vi "AlarmEngineModule.vi"(8 "error in (no error)":errorcluster, 9 "Shutdown Event":refnum<user-event>, 10 "Config":T1, 11 "ModuleID":string) -> (0 "error out":errorcluster)   [LabVIEW 2020, in "AlarmEngine.lvlib"]
uses:
  AlarmEngine.lvlib
  <vilib>/Utility/Data Type/Type Definitions/Data Type.ctl
  <vilib>/Utility/Data Type/NI_Data Type.lvlib
  eac3c09b-8ce1-4b18-8db3-0e6b686db002.vi
  <vilib>/Tag Engine/Types/SetRequest Cluster.ctl
  <vilib>/Tag Engine/Tag Engine Core.lvlib
  <vilib>/Tag Engine/Tag Expr/Tag Expr.lvclass
  fca5b91c-2f04-4d42-a9b6-24fda182e91a.vi
  cc66a33a-e2f7-4f32-842c-e417093018b7.vi
  <vilib>/Tag Engine/Tag/Tag.lvclass
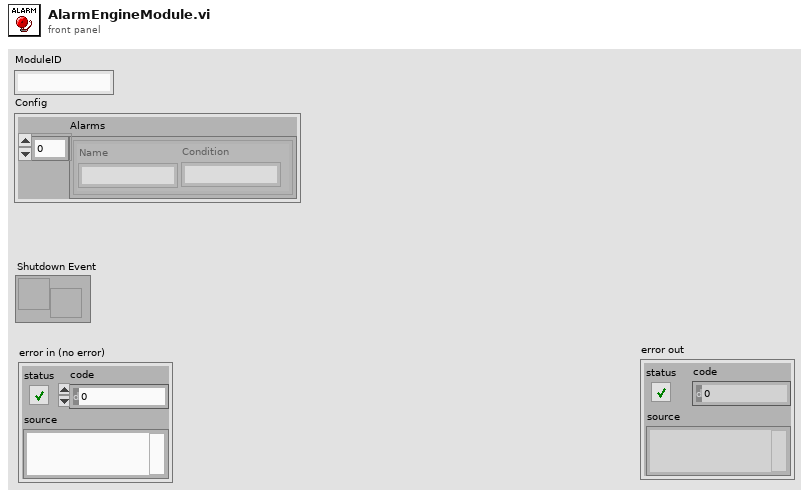
[diagram p1: front panel]
types:
  T1 = cluster{"Alarms":cluster{"Name":string, "Condition":string}[]}
  T2 = cluster{"Tag Refs":cluster{"ALARMS":refnum<data-value>[], "CONFIG":refnum<data-value>}, "Config":cluster{"Alarms":cluster{"Name":string, "Condition":string}[]}, "Conditions":refnum<class "Tag Expr.lvclass">[]}
  T3 = cluster{"ALARMS":refnum<data-value>[], "CONFIG":refnum<data-value>}
  T4 = cluster{"Config":cluster{"Alarms":cluster{"Name":string, "Condition":string}[]}, "Callback":refnum<notifier>}
  T5 = cluster{"Req Value":variant, "Callback":refnum<notifier>}
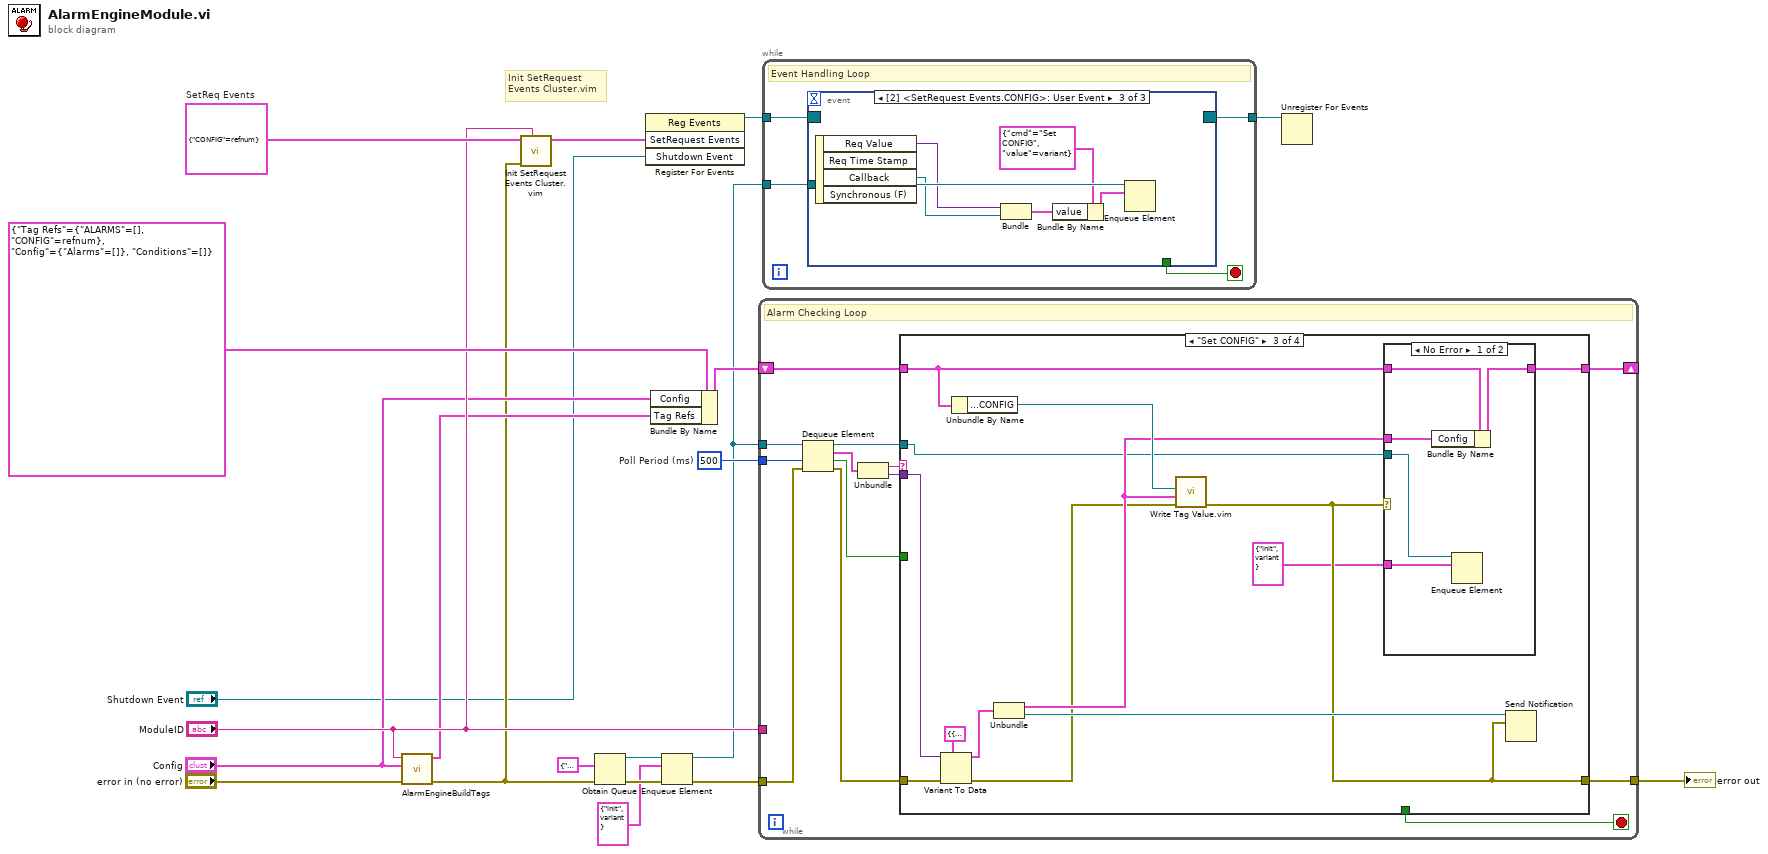
[diagram p0: block diagram]
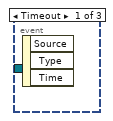
[diagram p2: hidden frame]
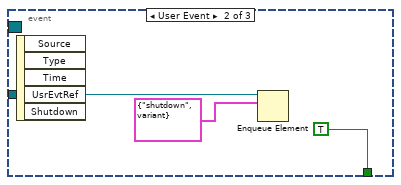
[diagram p3: hidden frame]
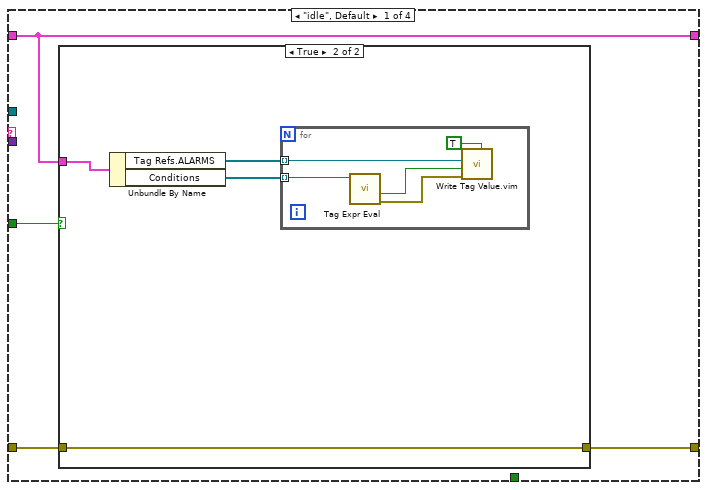
[diagram p4: hidden frame]
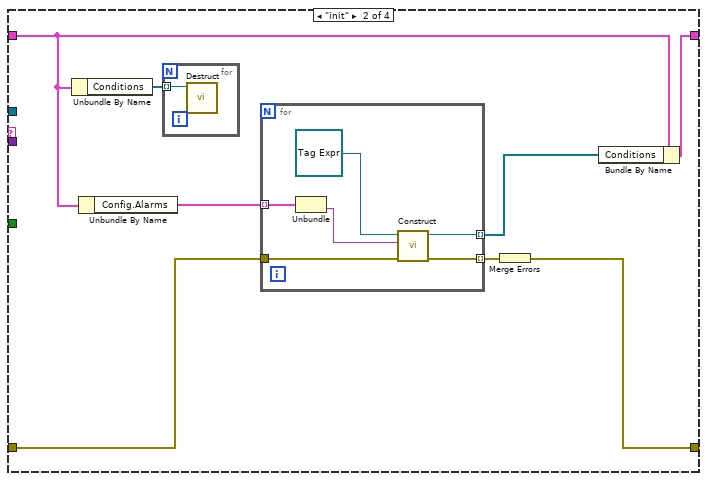
[diagram p6: hidden frame]
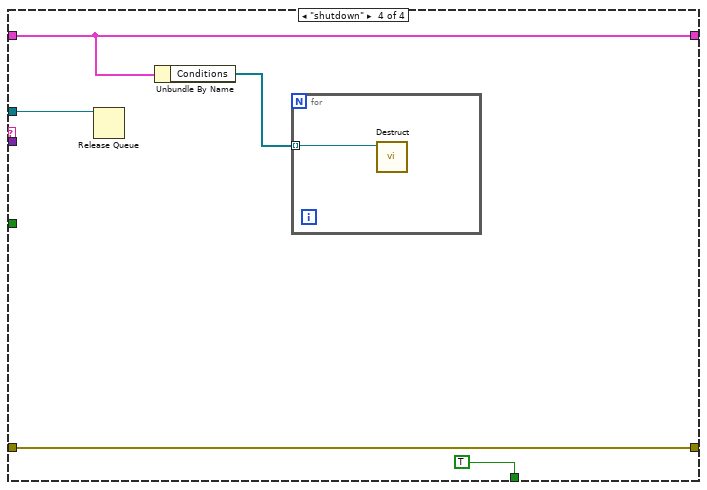
[diagram p8: hidden frame]
diagram:
  w7 = 500  # Poll Period (ms)
  w18 = cluster{"CONFIG":refnum<user-event>} {"CONFIG"=refnum}  # SetReq Events
  # "Init SetRequest\nEvents Cluster.vim"
  n1 = call "AlarmEngineBuildTags.vi"("error in (no error)"="error in (no error)", "Config"="Config", "ModuleID"="ModuleID") -> ("error out"=w9:errorcluster, "Tag Refs"=w10:T3)  [unwired: 7 in]
  n2 = call "Init SetRequest Events Cluster.vim"("Namespace"="ModuleID", "error in (no error)"=w9, "SetRequest Events in"=w18) -> ("SetRequest Events"=w17:cluster{"CONFIG":refnum<user-event>})  [unwired: 7 in, 1 out]
  n3 = Obtain Queue(element data type=cluster{"cmd":string, "value":variant} {"cmd"="", "value"=variant}, error in (no error)=w9) -> (queue out=w5:refnum<queue>, error out=w4:errorcluster)  [unwired: 3 in, 1 out]
  n4 = register-events(w17, "Shutdown Event") -> (reference out=w19:refnum<event-registration>)  [unwired: 2 in, 1 out]
  n5 = Bundle By Name(cluster=T2 {"Tag Refs"={"ALARMS"=[], "CONFIG"=refnum}, "Config"={"Alarms"=[]}, "Conditions"=[]}, "Config"="Config", "Tag Refs"=w10) -> (w8:T2)
  n6 = Enqueue Element(queue=w5, element=cluster{"cmd":string, "value":variant} {"cmd"="init", "value"=variant}, error in (no error)=w4) -> (queue out=w1:refnum<queue>, error out=w2:errorcluster)  [unwired: 1 in, 1 out]
  n7 = while {
    tunnel: "ModuleID" -> [_]
    tunnel: w2 -> [w33]
    shift-right: [w25] -> _
    shift-left: w8 -> [w32]
    tunnel: w1 -> [w29]
    tunnel: [w23] -> w15
    tunnel: w7 -> [w21]
    stop <- w24 stop-if-true
    # "Alarm Checking Loop"
    n8 = Dequeue Element(queue=w29, timeout in ms (-1)=w21, error in (no error)=w33) -> (queue out=w30:refnum<queue>, element=w28:cluster{"cmd":string, "value":variant}, timed out?=w22:bool, error out=w31:errorcluster)
    n9 = Unbundle(w28) -> ("cmd"=w27:string, "value"=w26:variant)
    n10 = case shown="\"Set CONFIG\"" w27 {
      tunnel: w32 -> [w37 w52 w66 w83]
      tunnel: w31 -> [w35 w50 w75 w84]
      tunnel: w30 -> [_ _ w64 w85]
      tunnel: w26 -> [_ _ w74 _]
      tunnel: [w37 w53 w70 w83] -> w25
      tunnel: [_ _ _ TRUE] -> w24
      tunnel: [w34 w48 w65 w84] -> w23
      tunnel: w22 -> [w36 _ _ _]
      frame "idle", Default {
        n11 = case shown="True" w36 {
          tunnel: w37 -> [_ w42]
          tunnel: w35 -> [w38 w39]
          tunnel: [w38 w39] -> w34
          frame False {
          }
          frame True {
            n12 = Unbundle By Name(w42) -> ("Tag Refs.ALARMS"=w40:refnum<data-value>[], "Conditions"=w41:refnum<class "Tag Expr.lvclass">[])
            n13 = for {
              tunnel: w41 -> [w47] mode=indexing
              tunnel: w40 -> [w46] mode=indexing
              n14 = call <vilib>:"Tag Expr Eval.vi"("Tag Expr in"=w47) -> ("error out"=w43:errorcluster, "Boolean Result"=w45:bool)  [unwired: 7 in, 2 out]
              n15 = call "Write Tag Value.vim"("IgnoreIfEqual (F)"=TRUE, "error in (no error)"=w43, "Value"=w45, "Tag Name(s)/Ref(s)"=w46) -> ()  [unwired: 6 in, 2 out]
            }
          }
        }
      }
      frame "init" {
        n16 = Unbundle By Name(w52) -> ("Conditions"=w54:refnum<class "Tag Expr.lvclass">[])
        n17 = Unbundle By Name(w52) -> ("Config.Alarms"=w55:cluster{"Name":string, "Condition":string}[])
        n18 = for {
          tunnel: w54 -> [w56] mode=indexing
          n19 = call-dynamic "Destruct.vi"("muExpr in"=w56) -> ()  [unwired: 10 in, 1 out]
        }
        n20 = for {
          tunnel: w55 -> [w62] mode=indexing
          tunnel: [w59] -> w51 mode=indexing
          tunnel: w50 -> [w58]
          tunnel: [w57] -> w49 mode=indexing
          n21 = Unbundle(w62) -> ("Condition"=w60:string)  [unwired: 1 out]
          n22 = call-dynamic "Construct.vi"("error in (no error)"=w58, "Expression"=w60, "Tag Expr in"=refnum<class "Tag Expr.lvclass"> refnum) -> ("error out"=w57:errorcluster, "Tag Expr out"=w59:refnum<class "Tag Expr.lvclass">)  [unwired: 5 in, 2 out]
        }
        n23 = Merge Errors(w49) -> (w48:errorcluster)
        n24 = Bundle By Name(cluster=w52, "Conditions"=w51) -> (w53:T2)
      }
      frame "Set CONFIG" {
        n25 = Variant To Data(error in=w75, type=T4 {"Config"={"Alarms"=[]}, "Callback"=refnum}, Variant=w74) -> (data=w72:T4, error out=w67:errorcluster)
        n26 = Unbundle By Name(w66) -> ("Tag Refs.CONFIG"=w69:refnum<data-value>)
        n27 = Unbundle(w72) -> ("Config"=w68:T1, "Callback"=w71:refnum<notifier>)
        n28 = call "Write Tag Value.vim"("error in (no error)"=w67, "Value"=w68, "Tag Name(s)/Ref(s)"=w69) -> ("error out"=w65:errorcluster)  [unwired: 7 in, 1 out]
        n29 = case shown="No Error" w65 {
          tunnel: [w80 w81] -> w70
          tunnel: w68 -> [w79 _]
          tunnel: w66 -> [w78 w81]
          tunnel: w64 -> [w77 _]
          tunnel: cluster{"cmd":string, "value":variant} {"cmd"="init", "value"=variant} ("element") -> [w76 _]
          frame No Error {
            n30 = Bundle By Name(cluster=w78, "Config"=w79) -> (w80:T2)
            n31 = Enqueue Element(queue=w77, element=w76) -> ()  [unwired: 2 in, 3 out]
          }
          frame Error {
          }
        }
        n32 = Send Notification(notification=w65, notifier=w71) -> ()  [unwired: 1 in, 2 out]
      }
      frame "shutdown" {
        n33 = Release Queue(queue=w85) -> ()  [unwired: 2 in, 3 out]
        n34 = Unbundle By Name(w83) -> ("Conditions"=w82:refnum<class "Tag Expr.lvclass">[])
        n35 = for {
          tunnel: w82 -> [w87] mode=indexing
          n36 = call-dynamic "Destruct.vi"("muExpr in"=w87) -> ()  [unwired: 10 in, 1 out]
        }
      }
    }
  }
  "error out" <- w15
  n37 = while {
    tunnel: [w91] -> w20
    tunnel: w19 -> [w90]
    tunnel: w1 -> [w88]
    stop <- w89 stop-if-true
    # "Event Handling Loop"
    n38 = event shown="[2] <SetRequest Events.CONFIG>: User Event" {
      selector: w90 -> [_ _ _]
      dyn-events: [_ _ _] -> w91
      timeout: _ -> [_ _ _]
      tunnel: [_ TRUE _] -> w89
      tunnel: w88 -> [_ w93 w100]
      event Timeout {
        n39 = event-data() -> ()  [unwired: 1 in, 3 out]
      }
      event User Event {
        n40 = event-data() -> ()  [unwired: 1 in, 5 out]
        n41 = Enqueue Element(queue=w93, element=cluster{"cmd":string, "value":variant} {"cmd"="shutdown", "value"=variant}) -> ()  [unwired: 2 in, 3 out]
      }
      event User Event {
        n42 = event-data() -> ("Req Value"=w97:variant, "Callback"=w95:refnum<notifier>)  [unwired: 1 in, 2 out]
        n43 = Bundle("Req Value"=w97, "Callback"=w95) -> (w96:T5)  [unwired: 1 in]
        n44 = Bundle By Name(cluster=cluster{"cmd":string, "value":variant} {"cmd"="Set CONFIG", "value"=variant} ("element"), "value"=w96) -> (w98:cluster{"cmd":string, "value":variant})
        n45 = Enqueue Element(queue=w100, element=w98) -> ()  [unwired: 2 in, 3 out]
      }
    }
  }
  n46 = Unregister For Events(event registration refnum=w20) -> ()  [unwired: 1 in, 1 out]
